vi "Identify Cryo-Con.vi"(8 "Error In":errorcluster, 11 "VISA resource name":refnum<visa-resource-name>) -> (0 "Error Out":errorcluster, 1 "data string out":string, 2 "Cryo-con":bool, 3 "VISA resource name out":refnum<visa-resource-name>)   [LabVIEW 2018]
uses:
  f46bd5af-de24-4e9e-a8e8-95635435b45a.vi
  <vilib>/Utility/error.llb/Error Cluster From Error Code.vi
  GPIB/VISA  Send Receive.vi
  <vilib>/ErrorRing/Error Ring.xnode
panel:
  in  "Serial Configuration":cluster{"Baud Rate":u32}={"Baud Rate"=9600} {"Baud Rate" items=["300"=300, "600"=600, "1200"=1200, "2400"=2400, "4800"=4800, "9600"=9600, "19200"=19200]}
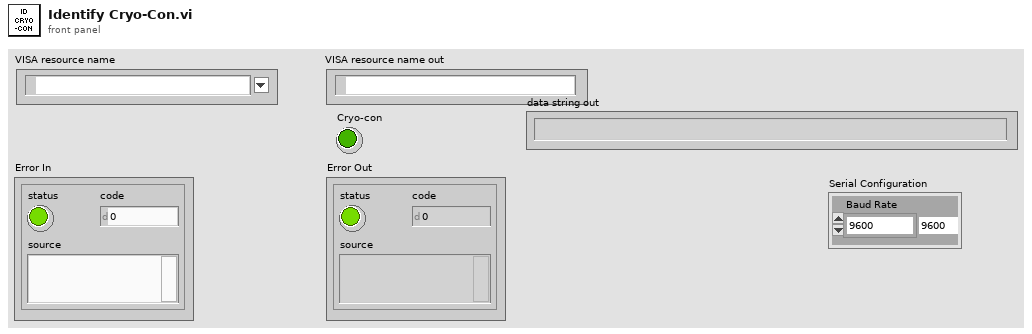
[diagram p1: front panel]
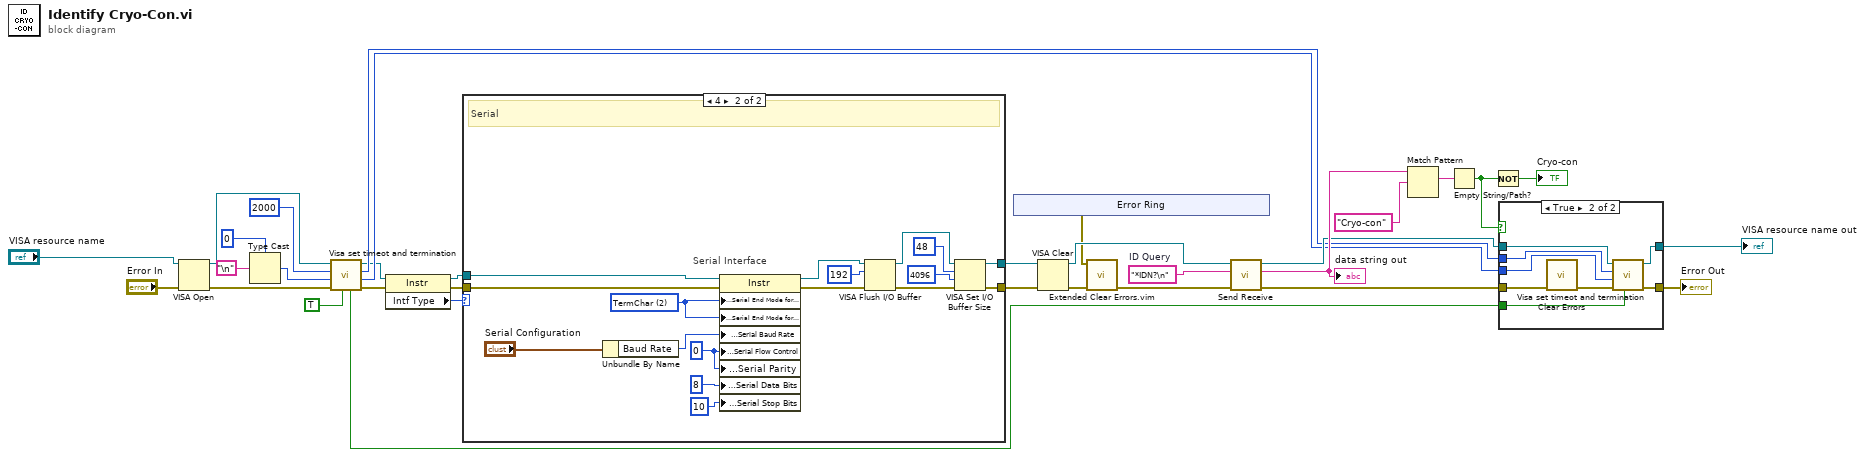
[diagram p0: block diagram]
diagram:
  w29 = "*IDN?\n"  # ID Query
  n1 = VISA Open(error in (no error)="Error In", VISA resource name="VISA resource name") -> (VISA resource name=w15:refnum<visa-resource-name>, error out=w13:errorcluster)  [unwired: 3 in]
  n2 = Type Cast(type=u8 0, x="\n" ("Line Feed Constant")) -> (*(type *) &x=w10:u8)
  n3 = call "Visa set timeot and termination.vi"("Termination Character Enable"=TRUE ("Message Based Settings:Termination Character Enable"), "error in (no error)"=w13, "Termination Character"=w10, "Timeout Value"=u32 2000 ("General Settings:Timeout Value"), "VISA resource name"=w15) -> ("error out"=w14:errorcluster, "Old Termination Character"=w8:u8, "Old Timeout Value"=w9:u32, "VISA resource name out"=w5:refnum<visa-resource-name>, "Old Termination Character Enable"=w7:bool)  [unwired: 2 in]
  n4 = property class="Instr"(reference=w5, error in=w14) -> (reference out=w4:refnum<visa-resource-name>, error out=w6:errorcluster, "Intf Type"=w3:u16)
  n5 = case shown="4" w3 {
    tunnel: [w34 w49] -> w17
    tunnel: [w35 w46] -> w16
    tunnel: w4 -> [w34 w51]
    tunnel: w6 -> [w35 w52]
    frame 0, Default {
      # "TCP/IP uses end-of-line char of \\n to terminate reads"
      # "GPIB and TCP/IP Interfaces"
    }
    frame 4 {
      w38 = u16 0
      w41 = u16 2 items=["None", "LastBit", "TermChar"] ("Serial Settings:Serial End Mode for Reads")
      # "Serial Interface"
      # "Serial"
      n6 = Unbundle By Name("Serial Configuration") -> ("Baud Rate"=w40:u32)
      n7 = property class="Instr"(reference=w51, error in=w52, "Serial Settings:Serial End Mode for Reads"=w41, "Serial Settings:Serial End Mode for Writes"=w41, "Serial Settings:Serial Baud Rate"=w40, "Serial Settings:Serial Flow Control"=w38, "Serial Settings:Serial Parity"=w38, "Serial Settings:Serial Data Bits"=u16 8, "Serial Settings:Serial Stop Bits"=u16 10) -> (reference out=w45:refnum<visa-resource-name>, error out=w48:errorcluster)
      n8 = VISA Flush I/O Buffer(VISA resource name=w45, mask (16)=u16 192, error in (no error)=w48) -> (VISA resource name out=w50:refnum<visa-resource-name>, error out=w47:errorcluster)
      n9 = VISA Set I/O Buffer Size(VISA resource name=w50, mask (16)=u16 48, size (4096)=u32 4096 ("size (0)"), error in (no error)=w47) -> (VISA resource name out=w49:refnum<visa-resource-name>, error out=w46:errorcluster)
    }
  }
  n10 = xnode "Error Ring"() -> ("error out"=w1:errorcluster)
  n11 = VISA Clear(VISA resource name=w17, error in (no error)=w16) -> (VISA resource name out=w19:refnum<visa-resource-name>, error out=w18:errorcluster)
  n12 = call "Extended Clear Errors.vim"("Error In"=w18, "specific error code to clear (0: all)"=w1) -> ("Error Out"=w2:errorcluster)  [unwired: 7 in, 2 out]
  n13 = call-poly "Send Receive.vi"("error in (no error)"=w2, "data string in"=w29, "VISA Resource Name"=w19) -> ("error out"=w23:errorcluster, "data string out"=w28:string, "VISA Resource Name Out"=w22:refnum<visa-resource-name>)  [unwired: 6 in]
  "data string out" <- w28
  n14 = Match Pattern(string=w28, regular expression="Cryo-con") -> (match substring=w26:string)  [unwired: 1 in, 3 out]
  n15 = Empty String/Path?(string/path=w26) -> (empty?=w24:bool)
  n16 = Not(x=w24) -> (.not. x?=→"Cryo-con":bool)
  n17 = case shown="True" w24 {
    tunnel: w23 -> [w54 w62]
    tunnel: w22 -> [w53 w61]
    tunnel: w9 -> [_ w59]
    tunnel: w7 -> [_ w58]
    tunnel: w8 -> [_ w57]
    tunnel: [w54 w55] -> w21
    tunnel: [w53 w60] -> w20
    frame False {
    }
    frame True {
      n18 = call <vilib>:"Clear Errors.vi"("error in (no error)"=w62) -> ("error out"=w56:errorcluster)  [unwired: 5 in, 1 out]
      n19 = call "Visa set timeot and termination.vi"("Termination Character Enable"=w58, "error in (no error)"=w56, "Termination Character"=w57, "Timeout Value"=w59, "VISA resource name"=w61) -> ("error out"=w55:errorcluster, "VISA resource name out"=w60:refnum<visa-resource-name>)  [unwired: 2 in, 3 out]
    }
  }
  "VISA resource name out" <- w20
  "Error Out" <- w21
